vi "tear_down.vi"(8 "error in (no error)":errorcluster, 11 "heat_board_control in":refnum<class "heat_board_control.lvclass">) -> (0 "error out":errorcluster, 3 "heat_board_control out":refnum<class "heat_board_control.lvclass">)   [LabVIEW 2015, in "heat_board_control.lvclass"]
uses:
  heat_board_control.lvclass
  <vilib>/Utility/error.llb/DialogType.ctl
  <vilib>/ULx/Write.llb/ULx Write (Analog 1D DBL 1Chan 1Samp).vi
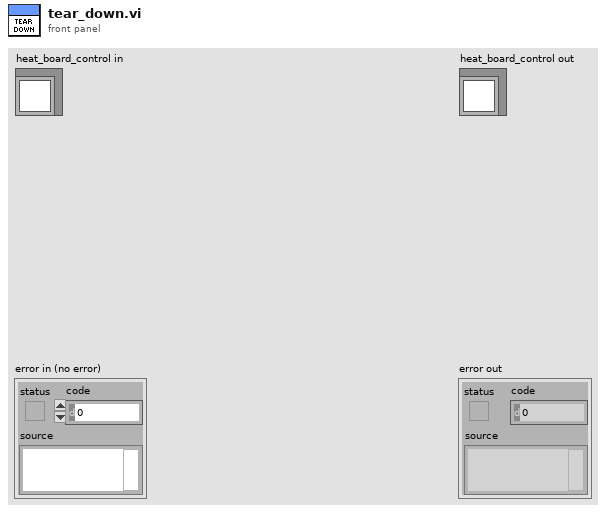
[diagram p1: front panel]
types:
  T1 = typedef "DialogType.ctl" = u16
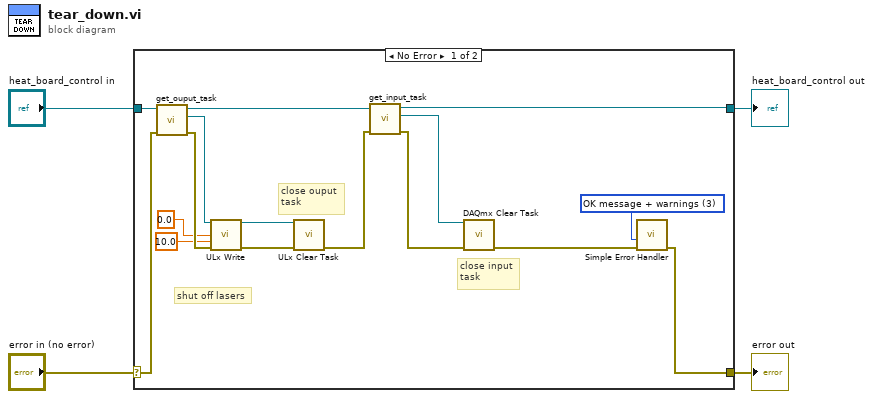
[diagram p0: block diagram]
diagram:
  n1 = case shown="No Error" "error in (no error)" {
    selector: "error in (no error)" -> [w15 w22]
    tunnel: [w19 w22] -> w3
    tunnel: [w13 w21] -> w1
    tunnel: "heat_board_control in" -> [w17 w21]
    frame No Error {
      w20 = T1 3 items=["no dialog", "OK message", "continue or stop message", "OK message + warnings", "continue/stop + warnings"] ("type of dialog (OK msg:1)")
      # "shut off lasers"
      # "close input\ntask"
      # "close ouput\ntask"
      n2 = call-dynamic "get_ouput_task.vi"("error in (no error)"=w15, "heat_board_control in"=w17) -> ("error out"=w10:errorcluster, "output task out"=w8:refnum<k24>, "heat_board_control out"=w16:refnum<class "heat_board_control.lvclass">)  [unwired: 7 in]
      n3 = call-poly <vilib>:"ULx Write.vi"("task in"=w8, "data"=0.0, "timeout"=10.0, "error in"=w10) -> ("task out"=w7:refnum<k24>, "error out"=w9:errorcluster)  [unwired: 9 in, 1 out]
      n4 = call <vilib>:"ULx Clear Task.vi"("task in"=w7, "error in"=w9) -> ("error out"=w12:errorcluster)  [unwired: 13 in]
      n5 = call-dynamic "get_input_task.vi"("error in (no error)"=w12, "heat_board_control in"=w16) -> ("error out"=w11:errorcluster, "input task out"=w14:refnum<k21>, "heat_board_control out"=w13:refnum<class "heat_board_control.lvclass">)  [unwired: 7 in]
      n6 = call <vilib>:"DAQmx Clear Task.vi"("task in"=w14, "error in"=w11) -> ("error out"=w18:errorcluster)  [unwired: 13 in]
      n7 = call <vilib>:"Simple Error Handler.vi"("type of dialog (OK msg:1)"=w20, "error in (no error)"=w18) -> ("error out"=w19:errorcluster)  [unwired: 3 in, 4 out]
    }
    frame Error {
    }
  }
  "error out" <- w3
  "heat_board_control out" <- w1
